vi "CAN Report Log.vi"(8 "error in (no error)":errorcluster, 11 "Socket":i16) -> (0 "error out":errorcluster, 2 "Log?":bool, 3 "refnum out":refnum<file>)   [LabVIEW 2023, in "LTT_TeststandSteptypes.lvlib"]
uses:
  LTT_TeststandSteptypes.lvlib
  HardwareAbstractionLayer_LVOOP/Report/Report_class/Control/Action FGV.ctl
  HardwareAbstractionLayer_LVOOP/Database/Database.lvclass
  HardwareAbstractionLayer_LVOOP/Report/Report_class/Report.lvclass
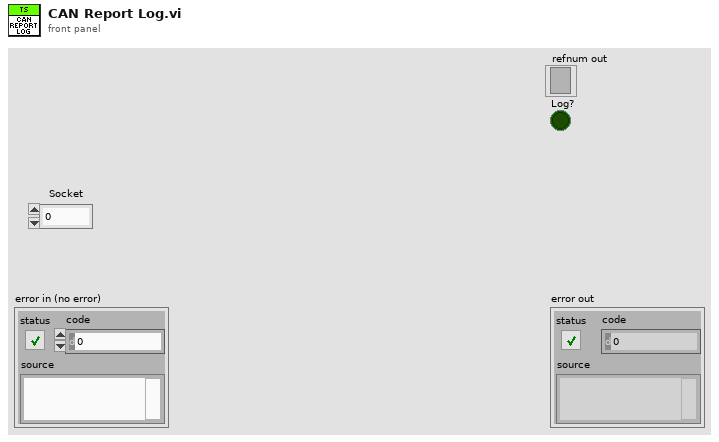
[diagram p1: front panel]
types:
  T1 = typedef "HardwareAbstractionLayer_LVOOP.lvlib/Report.lvclass/Action FGV.ctl" = enum16{"Init", "Set Project Name", "Set Product Name", "Set Product Varient", "Set Test Name", "Set Test Phase", "Set Test Description", "Set Temp Chamber Name", "Set Cycle Duration", "Set Current Cycle Number", "Set Schema", "Set Total No Of Cycle", "Set Current Test Mode", "Set All Data", "Get All Data"}
  T2 = typedef "HardwareAbstractionLayer_LVOOP.lvlib/Report.lvclass/Result FGV Data.ctl" = cluster{"Project Name":string, "Product Name":string, "Product Varient":string, "Test Name":string, "Test Phase":string, "Test Description":string, "Temp Chamber Name":string, "Schema":string, "Total No of Cycles":u32, "Current Cycle Number":u32, "Cycle Duration":u32, "Current Test Mode":string}
  T3 = enum16{"open", "replace", "create", "open or create", "replace or create", "replace or create with confirmation"}
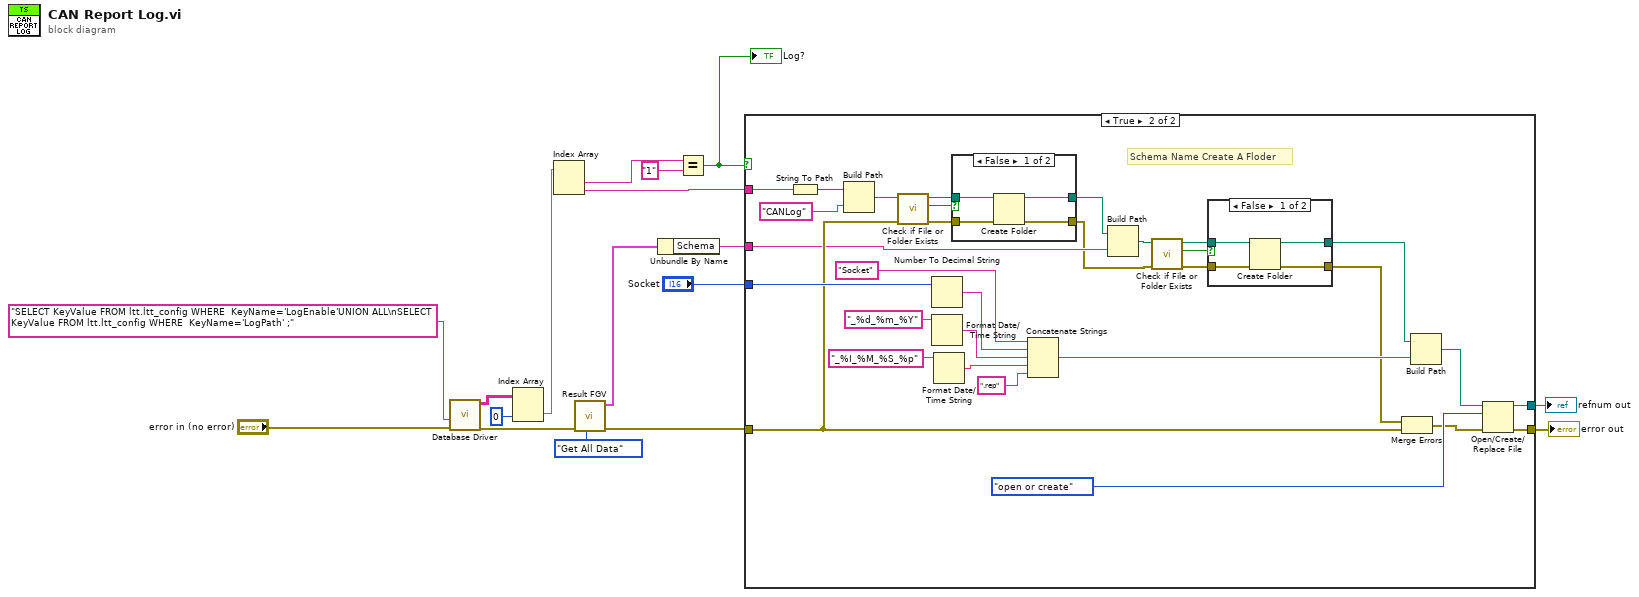
[diagram p0: block diagram]
diagram:
  n1 = call "Database Driver.vi"("error in"="error in (no error)", "SQL query"="SELECT KeyValue FROM ltt.ltt_config WHERE  KeyName='LogEnable'UNION ALL\nSELECT KeyValue FROM ltt.ltt_config WHERE  KeyName='LogPath' ;") -> ("error out"=w3:errorcluster, "data"=w16:string[][])  [unwired: 6 in, 2 out]
  n2 = Index Array(array=w16, index (col)=0 ("disabled index (col)")) -> (element=w15:string[])  [unwired: 1 in]
  n3 = Index Array(array=w15) -> (element #1=w14:string, element #2=w9:string)  [unwired: 2 in]
  n4 = call "Result FGV.vi"("Action(Get All Data)"=Action_FGV."Get All Data", "error in"=w3) -> ("error out"=w2:errorcluster, "Result FGV Data Out"=w4:T2)  [unwired: 8 in]
  n5 = Unbundle By Name(w4) -> ("Schema"=w1:string)
  n6 = Equal?(x=w14, y="1") -> (x = y?=w7:bool)
  "Log?" <- w7
  n7 = case shown="True" w7 {
    tunnel: w2 -> [w18 w32]
    tunnel: "Socket" -> [_ w40]
    tunnel: [w18 w39] -> w10
    tunnel: w9 -> [_ w38]
    tunnel: [_ w33] -> w8
    tunnel: w1 -> [_ w27]
    frame False {
    }
    frame True {
      # "Schema Name Create A Floder"
      n8 = String To Path(string=w38) -> (path=w36:path)
      n9 = Build Path(base path=w36, name or relative path="CANLog") -> (appended path=w35:path)
      n10 = call <vilib>:"Check if File or Folder Exists.vi"("error in (no error)"=w32, "path"=w35) -> ("error out"=w31:errorcluster, "file or folder exists?"=w30:bool, "dup path"=w29:path)  [unwired: 7 in]
      n11 = Number To Decimal String(number=w40) -> (decimal integer string=w47:string)  [unwired: 1 in]
      n12 = Format Date/Time String(time format string (%c)="_%d_%m_%Y") -> (date/time string=w46:string)  [unwired: 2 in]
      n13 = Format Date/Time String(time format string (%c)="_%I_%M_%S_%p") -> (date/time string=w45:string)  [unwired: 2 in]
      n14 = case shown="False" w30 {
        tunnel: w31 -> [w58 w60]
        tunnel: w29 -> [w59 w61]
        tunnel: [w57 w61] -> w26
        tunnel: [w56 w60] -> w21
        frame False {
          n15 = Create Folder(path (use dialog)=w59, error in=w58) -> (created path=w57:path, error out=w56:errorcluster)  [unwired: 1 in, 1 out]
        }
        frame True {
        }
      }
      n16 = Concatenate Strings("Socket", w47, w46, w45, ".rep" ("string")) -> (w43:string)
      n17 = Build Path(base path=w26, name or relative path=w27) -> (appended path=w22:path)
      n18 = call <vilib>:"Check if File or Folder Exists.vi"("error in (no error)"=w21, "path"=w22) -> ("error out"=w23:errorcluster, "file or folder exists?"=w24:bool, "dup path"=w25:path)  [unwired: 7 in]
      n19 = case shown="False" w24 {
        tunnel: w23 -> [w52 w54]
        tunnel: w25 -> [w53 w55]
        tunnel: [w51 w55] -> w20
        tunnel: [w50 w54] -> w19
        frame False {
          n20 = Create Folder(path (use dialog)=w53, error in=w52) -> (created path=w51:path, error out=w50:errorcluster)  [unwired: 1 in, 1 out]
        }
        frame True {
        }
      }
      n21 = Merge Errors(w19, w32) -> (w28:errorcluster)
      n22 = Build Path(base path=w20, name or relative path=w43) -> (appended path=w41:path)
      n23 = Open/Create/Replace File(file path (use dialog)=w41, error in=w28, operation (0:open)=T3."open or create") -> (refnum out=w33:refnum<file>, error out=w39:errorcluster)  [unwired: 3 in, 1 out]
    }
  }
  "error out" <- w10
  "refnum out" <- w8
